vi "UI_FP Open Close.vi"(8 "Error":errorcluster, 9 "State":T1(ring)=enum."Standard", 11 "Vi Ref (this Vi)":refnum<vi>) -> (0 "Error Out":errorcluster, 3 "Dup Ref Out":refnum<vi>)   [LabVIEW 2009]
doc: "Open or Closed the References front panel"
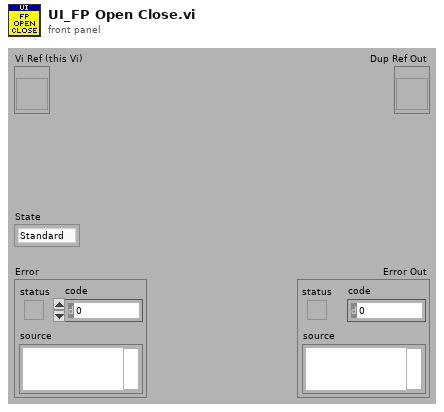
[diagram p1: front panel]
types:
  T1 = enum32{"Invalid", "Standard", "Closed", "Hidden", "Minimized", "Maximized"}
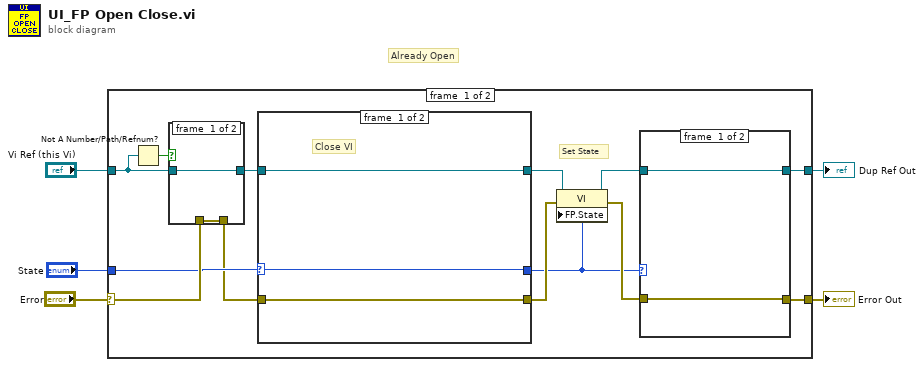
[diagram p0: block diagram]
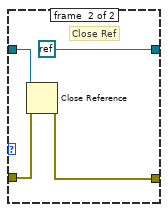
[diagram p2: hidden frame]
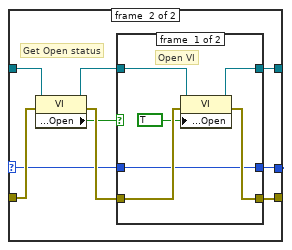
[diagram p3: hidden frame]
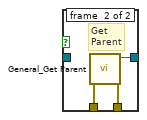
[diagram p5: hidden frame]
diagram:
  # "Already Open"
  n1 = case shown="No Error" "Error" {
    selector: "Error" -> [w16 w51]
    tunnel: "Vi Ref (this Vi)" -> [w17 w52]
    tunnel: [w14 w52] -> w4
    tunnel: [w15 w51] -> w3
    tunnel: "State" -> [w13 _]
    frame #0 {
      # "Set State"
      n2 = Not A Number/Path/Refnum?(number/path/refnum=w17) -> (NaN/Path/Refnum?=w18:bool)
      n3 = case shown="True" w18 {
        tunnel: [w47 w50] -> w12
        tunnel: w17 -> [w47 _]
        tunnel: w16 -> [w46 w49]
        tunnel: [w46 w48] -> w9
        frame #0 {
        }
        frame #1 {
          # "Get\nParent"
          n4 = call "General_Get Parent.vi"("Error In (no Error)"=w49) -> ("Error Out"=w48:errorcluster, "VI Refnum Out"=w50:refnum<vi>)  [unwired: 8 in, 1 out]
        }
      }
      n5 = case shown="Default" w13 {
        selector: w13 -> [w27 w29]
        tunnel: w12 -> [w26 w36]
        tunnel: [w26 w34] -> w11
        tunnel: [w27 w28] -> w6
        tunnel: w9 -> [w25 w33]
        tunnel: [w25 w31] -> w10
        frame #0 {
          # "Close VI"
        }
        frame #1 {
          # "Get Open status"
          n6 = property class="VI"(reference=w36, error in=w33) -> (reference out=w35:refnum<vi>, error out=w32:errorcluster, "Front Panel.Open"=w30:bool)
          n7 = case shown="False" w30 {
            tunnel: w35 -> [w42 w45]
            tunnel: [w41 w45] -> w34
            tunnel: w32 -> [w40 w43]
            tunnel: [w39 w43] -> w31
            tunnel: w29 -> [w38 w44]
            tunnel: [w38 w44] -> w28
            frame #0 {
              # "Open VI"
              n8 = property class="VI"(reference=w42, error in=w40, "Front Panel.Open"=TRUE ("Front Panel Window:Open")) -> (reference out=w41:refnum<vi>, error out=w39:errorcluster)
            }
            frame #1 {
              # "Already Open"
            }
          }
        }
      }
      n9 = property class="VI"(reference=w11, error in=w10, "FP.State"=w6) -> (reference out=w7:refnum<vi>, error out=w8:errorcluster)
      n10 = case shown="\"Invalid\", \"Closed\"" w6 {
        tunnel: [w19 w24] -> w15
        tunnel: [w20 refnum<k0> refnum] -> w14
        tunnel: w8 -> [w19 w22]
        tunnel: w7 -> [w20 w21]
        frame #0 {
        }
        frame #1 {
          # "Close Ref"
          n11 = Close Reference(reference=w21, error in (no error)=w22) -> (error out=w24:errorcluster)
        }
      }
    }
    frame #1 {
    }
  }
  "Dup Ref Out" <- w4
  "Error Out" <- w3
